vi "Get Taps.vi"(8 "error in (no error)":errorcluster, 11 "TLCamera reference in":refnum<k24>) -> (0 "error out":errorcluster, 2 "Taps":i32(ring) items=["SingleTap", "DualTap", "QuadTap"], 3 "TLCamera reference out":refnum<k24>)   [LabVIEW 2022 SP3]
uses:
  I:/.shortcut-targets-by-id/1riZacJd_1_jmKfGgrjDuP7KcecvMS3i2/Xiao research group/Programs/XYZRecorrection/Scientific Camera Interfaces/SDK/DotNet Toolkit/dlls/Managed_64_lib/Thorlabs.TSI.TLCamera.dll
  SDK/DotNet Toolkit/dlls/Managed_64_lib/Thorlabs.TSI.TLCamera.dll
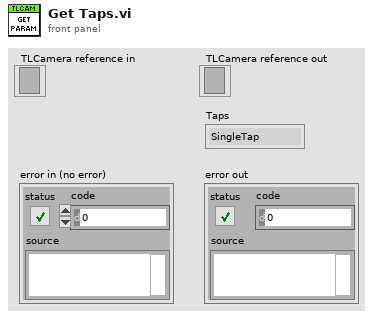
[diagram p1: front panel]
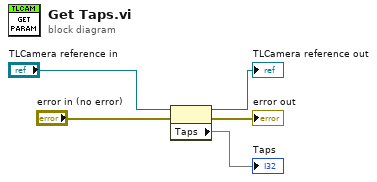
[diagram p0: block diagram]
diagram:
  n1 = property(reference="TLCamera reference in", error in="error in (no error)") -> (reference out=→"TLCamera reference out":refnum<k24>, error out=→"error out":errorcluster, "Taps"=→"Taps")
